vi "SeCrTs-Error handler RT.vi"(8 "error in":errorcluster, 11 "Message Queue":refnum<queue>) -> (0 "error out":errorcluster, 3 "Duq Message Queue":refnum<queue>)   [LabVIEW 2022 SP3]
uses:
  c8e64d7e-ce45-4cfd-9636-85734d5256d9.vi
  6ecc959c-78fe-438c-aec5-e12e03fb8790.vi
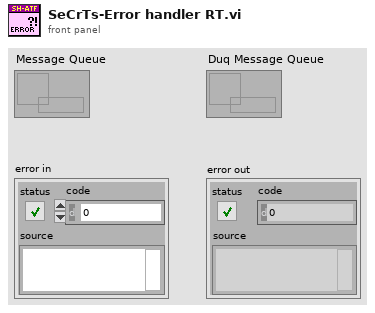
[diagram p1: front panel]
types:
  T1 = cluster{"Error Code":string, "Error Source":string}
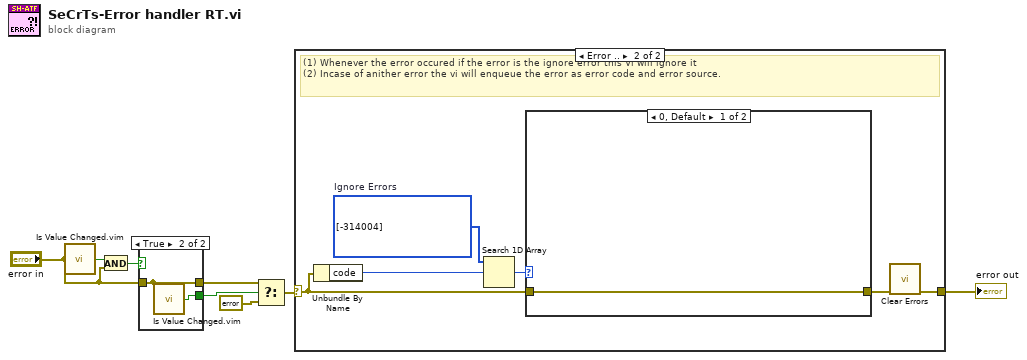
[diagram p0: block diagram]
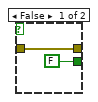
[diagram p2: hidden frame]
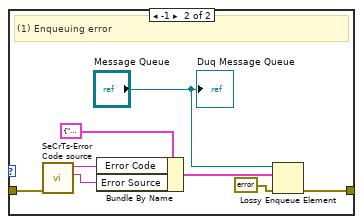
[diagram p4: hidden frame]
diagram:
  n1 = call "Is Value Changed.vim"("value"="error in") -> ("changed or first call?"=w5:bool)
  n2 = And(x=w5, y="error in") -> (x .and. y?=w1:bool)
  n3 = case shown="True" w1 {
    tunnel: "error in" -> [w9 w11]
    tunnel: [FALSE ("changed or first call?") w12] -> w3
    tunnel: [w9 w11] -> w2
    frame False {
    }
    frame True {
      n4 = call "Is Value Changed.vim"("value"=w11) -> ("changed or first call?"=w12:bool)
    }
  }
  n5 = Select(t=w2, s=w3, f=errorcluster {"status"=FALSE, "code"=0, "source"=""}) -> (s? t:f=w6:errorcluster)
  n6 = case shown="Error .." w6 {
    selector: w6 -> [w13 w16]
    tunnel: [w13 w14] -> w8
    frame No Error {
    }
    frame Error {
      w18 = i32[] [-314004]  # Ignore Errors
      # "(1) Whenever the error occured if the error is the ignore error this Vi will ignore it\n(2) Incase of anither error the vi will enqueue the error as error code and error source."
      n7 = Unbundle By Name(w16) -> ("code"=w19:i32)
      n8 = Search 1D Array(1D array=w18, element=w19) -> (index of element=w17:i32)  [unwired: 1 in]
      n9 = case shown="0, Default" w17 {
        tunnel: w16 -> [w20 w23]
        tunnel: [w20 w25] -> w15
        frame 0, Default {
        }
        frame -1 {
          # "(1) Enqueuing error"
          n10 = call "SeCrTs-Error Code source .vi"("error in (no error)"=w23) -> ("String"=w21:string, "String 2"=w22:string)  [unwired: 9 in]
          n11 = Bundle By Name(cluster=T1 {"Error Code"="", "Error Source"=""} ("element"), "Error Code"=w22, "Error Source"=w21) -> (w26:T1)
          n12 = Lossy Enqueue Element(queue="Message Queue", element=w26, error in (no error)=errorcluster {"status"=FALSE, "code"=0, "source"=""}) -> (error out=w25:errorcluster)  [unwired: 3 out]
          "Duq Message Queue" <- "Message Queue"
        }
      }
      n13 = call <vilib>:"Clear Errors.vi"("error in (no error)"=w15) -> ("error out"=w14:errorcluster)  [unwired: 5 in, 1 out]
    }
  }
  "error out" <- w8
